vi "Converted Data to Raw.vi"(0 "Data In":T1 {"CRC" format="%04x"; "Length" format="%02x"; "Command" format="%02x"; "Destination" format="%02x"; "Source" format="%02x"}, 11 "Error In":errorcluster) -> (4 "Raw Data Out":string, 15 "Error Out":errorcluster)   [LabVIEW 2016, in "GEA2_Toolkit.lvlib"]
uses:
  library/GEA2_Toolkit.lvlib
  type defs/Data Out.ctl
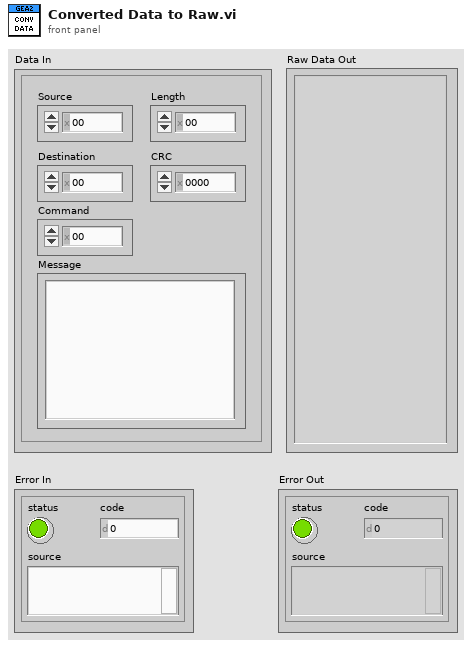
[diagram p1: front panel]
types:
  T1 = typedef "GEA2_Toolkit.lvlib/Data Out.ctl" = cluster{"Source":u8, "Destination":u8, "Command":u8, "Length":u8, "CRC":u16, "Message":string}
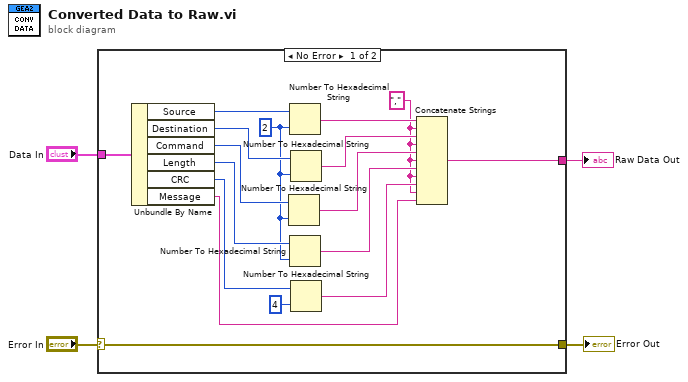
[diagram p0: block diagram]
diagram:
  n1 = case shown="No Error" "Error In" {
    selector: "Error In" -> [w21 w22]
    tunnel: [w21 w22] -> w3
    tunnel: "Data In" -> [w20 _]
    tunnel: [w7 _] -> w1
    frame No Error {
      w6 = i16 2 ("width (-)")
      w8 = ","
      n2 = Unbundle By Name(w20) -> ("Source"=w19:u8, "Destination"=w17:u8, "Command"=w16:u8, "Length"=w15:u8, "CRC"=w14:u16, "Message"=w9:string)
      n3 = Number To Hexadecimal String(1:w6, 2:w16) -> (0:w12:string)
      n4 = Number To Hexadecimal String(1:w6, 2:w19) -> (0:w18:string)
      n5 = Number To Hexadecimal String(1:w6, 2:w15) -> (0:w11:string)
      n6 = Number To Hexadecimal String(1:w6, 2:w17) -> (0:w13:string)
      n7 = Number To Hexadecimal String(1:i16 4 ("width (-)"), 2:w14) -> (0:w10:string)
      n8 = Concatenate Strings(w18, w8, w13, w8, w12, w8, w11, w8, w10, w8, w9) -> (w7:string)
    }
    frame Error {
    }
  }
  "Error Out" <- w3
  "Raw Data Out" <- w1
